vi "Refresh Channel Names and Defaults.vi"(8 "error in (no error)":errorcluster, 10 "engine configuration in":refnum<class "engine configuration.lvclass">, 11 "SHM configuration in":refnum<class "Shared Memory configuration.lvclass">) -> (0 "error out":errorcluster, 2 "engine configuration out":refnum<class "engine configuration.lvclass">, 3 "SHM configuration out":refnum<class "Shared Memory configuration.lvclass">)   [LabVIEW 2013, in "Shared Memory editor node.lvclass"]
uses:
  Shared Memory editor node.lvclass
  <vilib>/NI/Module Execution Interface/Engine Configuration/engine configuration.lvclass
  module/configuration/Shared Memory configuration.lvclass
  <vilib>/NI/Configuration Framework/serializable configuration/NISE_CEF_serializable configuration.lvclass/NISE_CEF_serializable configuration.ctl
  module/configuration/Shared Memory configuration.lvclass/Shared Memory configuration.ctl
  <vilib>/NI/Tag Bus/tag/tag descriptor.lvclass/tag descriptor.ctl
  <vilib>/NI/Tag Bus/tag/write tag name.vi
  <vilib>/NI/Configuration Framework/serializable configuration/Read UID.vi
  module/configuration/Read Lines.vi
  <vilib>/Utility/LVClass/Get LV Class Name.vi
  <vilib>/NI/Configuration Framework/error generator/NISE_error generator.vi
  <vilib>/NI/Tag Bus Module Framework/channel/TBM channel.lvclass
  <vilib>/NI/Tag Bus/tag/tag descriptor.lvclass
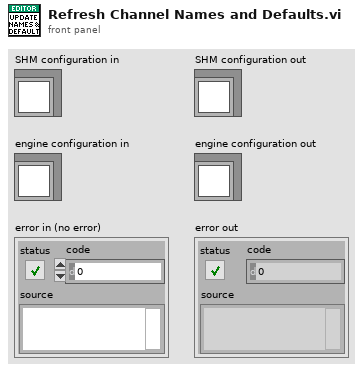
[diagram p1: front panel]
types:
  T1 = typedef "Shared Memory configuration.lvclass/Line.ctl" = cluster{"channel":refnum<class "TBM channel.lvclass">}
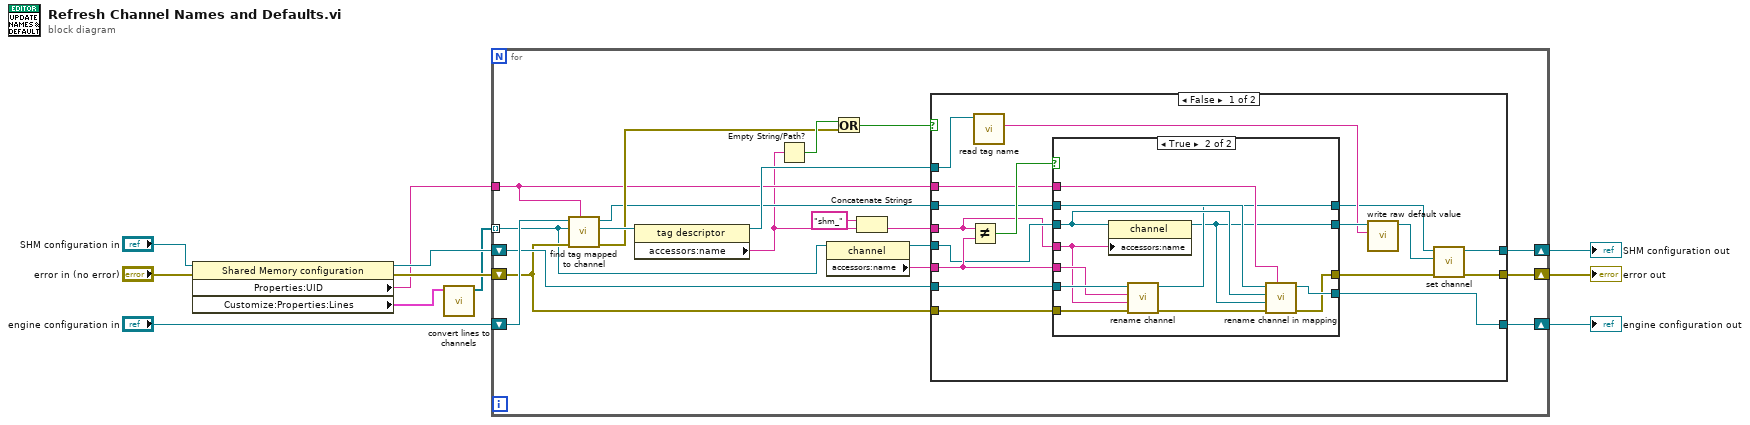
[diagram p0: block diagram]
diagram:
  n1 = property class="Shared Memory configuration"(reference="SHM configuration in", error in="error in (no error)") -> (reference out=w8:refnum<class "Shared Memory configuration.lvclass">, error out=w9:errorcluster, "Properties:UID"=w2:string, "Customize:Properties:Lines"=w4:T1[])
  n2 = call "convert lines to channels.vi"("Lines in"=w4) -> ("channels out"=w3:refnum<class "TBM channel.lvclass">[])  [unwired: 9 in, 1 out]
  n3 = for {
    tunnel: w3 -> [w15] mode=indexing
    tunnel: w2 -> [w20]
    shift-right: [w18] -> w5
    shift-left: w9 -> [w19]
    shift-right: [w17] -> w7
    shift-left: w8 -> [w22]
    shift-right: [w16] -> w6
    shift-left: "engine configuration in" -> [w30]
    n4 = call <vilib>:"find tag mapped to channel.vi"("owner"=w20, "error in"=w19, "channel"=w15, "engine configuration in"=w30) -> ("error out"=w27:errorcluster, "tag"=w29:refnum<class "tag descriptor.lvclass">, "engine configuration out"=w21:refnum<class "engine configuration.lvclass">)  [unwired: 5 in]
    n5 = property class="tag descriptor"(reference=w29) -> (reference out=w25:refnum<class "tag descriptor.lvclass">, "accessors:name"=w14:string)  [unwired: 1 in, 1 out]
    n6 = Empty String/Path?(string/path=w14) -> (empty?=w28:bool)
    n7 = property class="channel"(reference=w15) -> (reference out=w23:refnum<class "TBM channel.lvclass">, "accessors:name"=w24:string)  [unwired: 1 in, 1 out]
    n8 = Or(x=w28, y=w27) -> (x .or. y?=w26:bool)
    n9 = Concatenate Strings("shm_" ("string"), w14) -> (w13:string)
    n10 = case shown="False" w26 {
      tunnel: w25 -> [w47 _]
      tunnel: w13 -> [w42 _]
      tunnel: w24 -> [w44 _]
      tunnel: w23 -> [w43 _]
      tunnel: w22 -> [w45 w65]
      tunnel: w21 -> [w41 w66]
      tunnel: w20 -> [w40 _]
      tunnel: w19 -> [w39 w64]
      tunnel: [w33 w64] -> w18
      tunnel: [w32 w65] -> w17
      tunnel: [w31 w66] -> w16
      frame False {
        n11 = Not Equal?(x=w42, y=w44) -> (x != y?=w46:bool)
        n12 = call <vilib>:"read tag name.vi"("system tag in"=w47) -> ("name"=w37:string)  [unwired: 8 in, 2 out]
        n13 = case shown="True" w46 {
          tunnel: w45 -> [w51 w63]
          tunnel: w44 -> [_ w62]
          tunnel: w43 -> [w49 w58]
          tunnel: w42 -> [_ w61]
          tunnel: w41 -> [w50 w60]
          tunnel: w40 -> [_ w59]
          tunnel: [w51 w56] -> w36
          tunnel: [w50 w55] -> w31
          tunnel: [w48 w54] -> w34
          tunnel: w39 -> [w48 w53]
          tunnel: [w49 w52] -> w38
          frame False {
          }
          frame True {
            n14 = property class="channel"(reference=w58, "accessors:name"=w61) -> (reference out=w52:refnum<class "TBM channel.lvclass">)  [unwired: 1 in, 1 out]
            n15 = call "rename channel.vi"("error in"=w53, "new name"=w61, "old name"=w62, "SHM configuration in"=w63) -> ("error out"=w57:errorcluster, "SHM configuration out"=w56:refnum<class "Shared Memory configuration.lvclass">)  [unwired: 6 in]
            n16 = call <vilib>:"rename channel in mapping.vi"("owner ID"=w59, "error in"=w57, "new channel"=w52, "old channel"=w58, "engine configuration in"=w60) -> ("error out"=w54:errorcluster, "engine configuration out"=w55:refnum<class "engine configuration.lvclass">)  [unwired: 5 in]
          }
        }
        n17 = call <vilib>:"write raw default value.vi"("raw default"=w37, "system tag in"=w38) -> ("system tag out"=w35:refnum<class "TBM channel.lvclass">)  [unwired: 8 in, 1 out]
        n18 = call "set channel.vi"("error in"=w34, "TBM channel in"=w35, "SHM configuration in"=w36) -> ("error out"=w33:errorcluster, "SHM configuration out"=w32:refnum<class "Shared Memory configuration.lvclass">)  [unwired: 7 in]
      }
      frame True {
      }
    }
  }
  "engine configuration out" <- w6
  "SHM configuration out" <- w7
  "error out" <- w5
